vi "IO_Dataq_Read_Measurement.vi"(8 "error in (no error)":errorcluster, 10 "Num Chan":i32, 11 "VISA Refnum in":refnum<visa-resource-name>) -> (0 "error out":errorcluster, 1 "Outputs":dbl[](array[numeric]), 2 "Waveform Chart":dbl[][](graph)=[[3.57208251953125], [3.55621337890625], [3.55621337890625], [3.55621337890625], [3.56170654296875], [3.56689453125], [3.56170654296875], [3.56170654296875], [3.55621337890625], [3.56170654296875], [3.56170654296875], [3.55621337890625], [3.56689453125], [3.56170654296875], [3.55621337890625], [3.56170654296875], [3.56689453125], [3.56170654296875], [3.56170654296875], [3.56689453125], [3.56170654296875], [3.57208251953125], [3.56170654296875], [3.57208251953125], [3.56170654296875], [3.55621337890625], [3.55621337890625], [3.56689453125], [3.551025390625], [3.56170654296875], [3.55621337890625], [3.56170654296875]], 3 "VISA Refnum out":refnum<visa-resource-name>, 4 "Bytes at Port":u32)   [LabVIEW 2024]
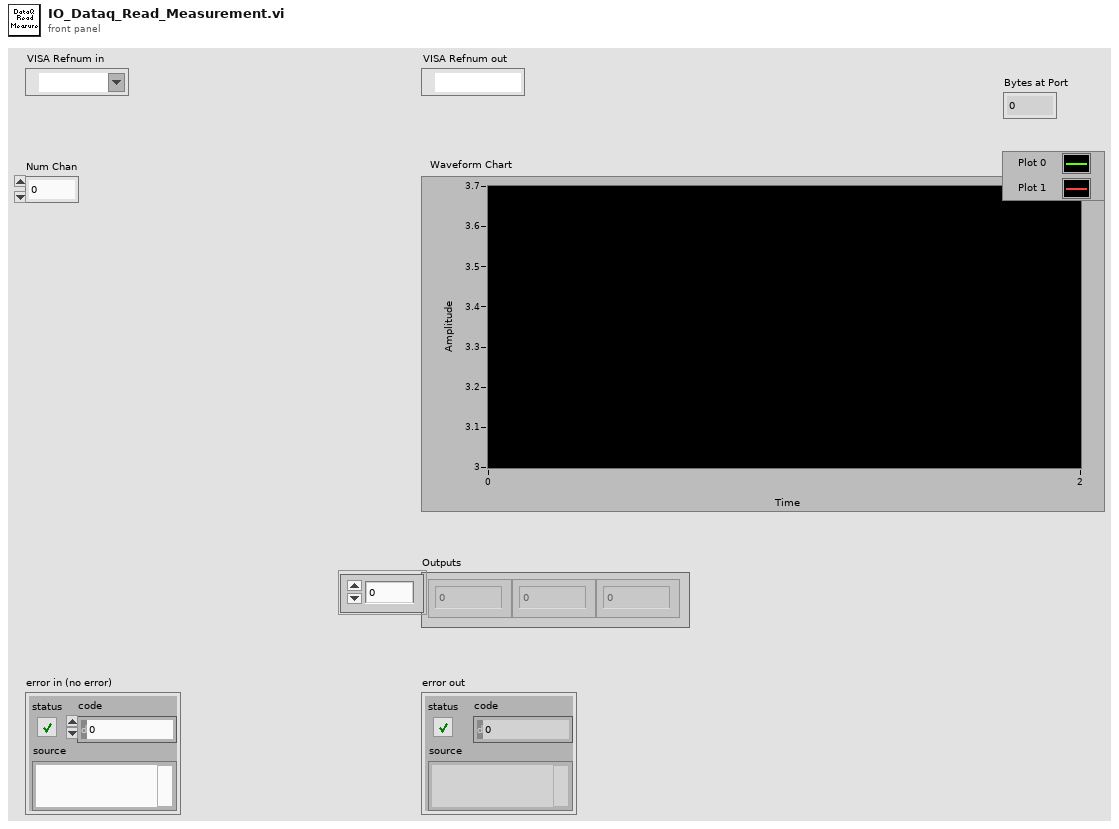
[diagram p1: front panel]
types:
  T1 = enum16{"big-endian, network order", "native, host order", "little-endian"}
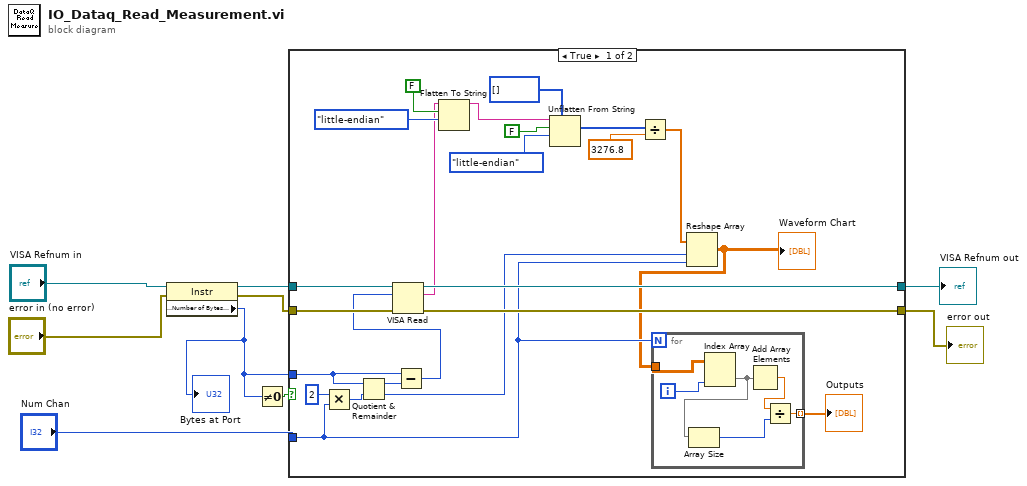
[diagram p0: block diagram]
diagram:
  n1 = property class="Instr"(reference="VISA Refnum in", error in="error in (no error)") -> (reference out=w4:refnum<visa-resource-name>, error out=w6:errorcluster, "Serial Settings:Number of Bytes at Serial Port"=w7:u32)
  "Bytes at Port" <- w7
  n2 = Not Equal To 0?(x=w7) -> (x != 0?=w8:bool)
  n3 = case shown="True" w8 {
    tunnel: [w31 w39] -> w1
    tunnel: w6 -> [w32 w40]
    tunnel: [w27 w40] -> w2
    tunnel: w4 -> [w14 w39]
    tunnel: w7 -> [w13 _]
    tunnel: "Num Chan" -> [w11 _]
    frame True {
      n4 = Multiply(x=2, y=w11) -> (x*y=w15:i32)
      n5 = Quotient & Remainder(x=w13, y=w15) -> (x-y*floor(x/y)=w29:u32, floor(x/y)=w17:u32)
      n6 = Subtract(x=w13, y=w29) -> (x-y=w28:u32)
      n7 = VISA Read(VISA resource name=w14, byte count=w28, error in (no error)=w32) -> (VISA resource name out=w31:refnum<visa-resource-name>, read buffer=w21:string, error out=w27:errorcluster)  [unwired: 1 out]
      n8 = Flatten To String(anything=w21, prepend array or string size? (T)=FALSE, byte order (0:big-endian, network order)=T1."little-endian") -> (data string=w22:string)  [unwired: 1 in, 2 out]
      n9 = Unflatten From String(type=i16[] [], binary string=w22, data includes array or string size? (T)=FALSE, byte order (0:big-endian, network order)=T1."little-endian") -> (value=w20:i16[])  [unwired: 1 in, 2 out]
      n10 = Divide(x=w20, y=3276.8) -> (x/y=w18:dbl[])
      n11 = Reshape Array(w18, w17, w11) -> (w10:dbl[][])
      "Waveform Chart" <- w10
      n12 = for {
        N: w11 -> [_]
        tunnel: w10 -> [w38]
        tunnel: [w35] -> w12 mode=indexing
        i -> [w33]
        n13 = Index Array(array=w38, index (col)=w33) -> (element=w34:dbl[])  [unwired: 1 in]
        n14 = Array Size(array=w34) -> (size(s)=w36:i32)
        n15 = Add Array Elements(numeric array=w34) -> (sum=w37:dbl)
        n16 = Divide(x=w37, y=w36) -> (x/y=w35:dbl)
      }
      "Outputs" <- w12
    }
    frame False {
    }
  }
  "error out" <- w2
  "VISA Refnum out" <- w1
